vi "ep_Check Overlap.vi"(8 "error in (no error)":errorcluster, 11 "% overlap":dbl) -> (0 "error out":errorcluster)   [LabVIEW 2014, in "NI_EP_Motor Monitoring.lvlib"]
uses:
  <vilib>/addons/Electrical Power/Motor Monitoring/NI_EP_Motor Monitoring.lvlib
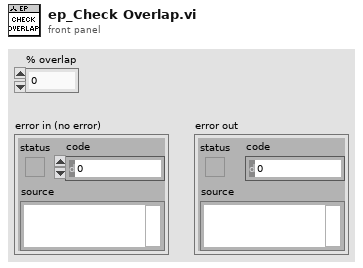
[diagram p1: front panel]
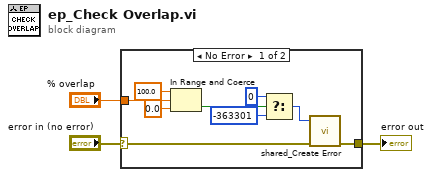
[diagram p0: block diagram]
diagram:
  n1 = case shown="No Error" "error in (no error)" {
    selector: "error in (no error)" -> [w6 w13]
    tunnel: "% overlap" -> [w7 _]
    tunnel: [w5 w13] -> w1
    frame No Error {
      n2 = In Range and Coerce(upper limit=100.0, x=w7, lower limit=0.0) -> (In Range?=w12:bool)  [unwired: 1 out]
      n3 = Select(t=0 ("error code (0)"), s=w12, f=-363301 ("error code (0)")) -> (s? t:f=w4:i32)
      n4 = call <vilib>:"shared_Create Error.vi"("error in (no error)"=w6, "error code (0)"=w4) -> ("error out"=w5:errorcluster)  [unwired: 9 in]
    }
    frame Error {
    }
  }
  "error out" <- w1
